vi "LEP_RV_BuildSpec_CommOptionsDlg.vi"(8 "error in (no error)":errorcluster, 10 "page sync rendezvous":T3, 11 "Close Event":refnum<user-event>) -> ()   [LabVIEW 2011]
doc: "Specifies TCP/IP options."
uses:
  resource/dialog/PreferencesDialog/optionsFrame_EventData1.ctl
  resource/dialog/PreferencesDialog/optionsFrame_PageInitData.ctl
  <vilib>/Platform/EmbProject/Plugins/utilities/LEP_Utilities_GetSetProjectData_Variant.vi
  <vilib>/Platform/EmbProject/Plugins/utilities/LEP_Utilities_GetSetProjectData_U32.vi
panel:
  out "Build settings conflicts":i32(listbox)=1
  in  "Target serial port":u16(ring) items=["0", "1", "2", "3"]
  in  "Console output":T1(radio)
  in  "MAC in target memory":bool
  in  "Secondary DNS":string
  in  "Primary DNS":string
  in  "MAC address":string
  in  "Target name":string
  in  "Gateway":string
  in  "Subnet mask":string
  in  "IP address":string
  in  "Use DHCP":bool
  in  "Page VI Init Data":T2
  in  "error msg format string":string="There was a problem applying the options from the %s category. The error message is \"%s.\""
  # "Console Output"
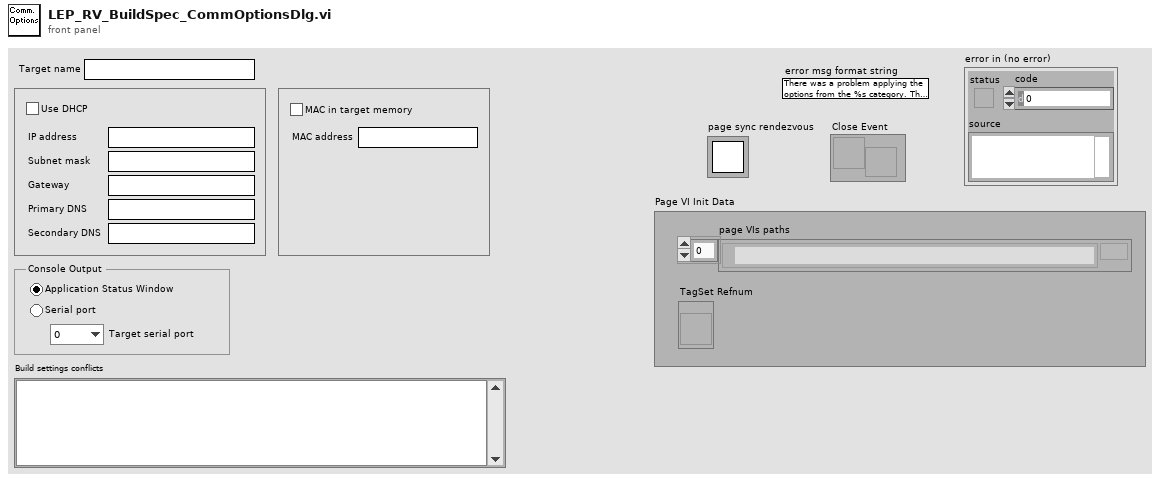
[diagram p1: front panel]
types:
  T1 = enum32{"Application Status Window", "Serial port"}
  T2 = typedef "optionsFrame_PageInitData.ctl" = cluster{"page VIs paths":path[], "TagSet Refnum":refnum<vi>}
  T3 = typedef "Rendezvous RefNum" = refnum<k1>
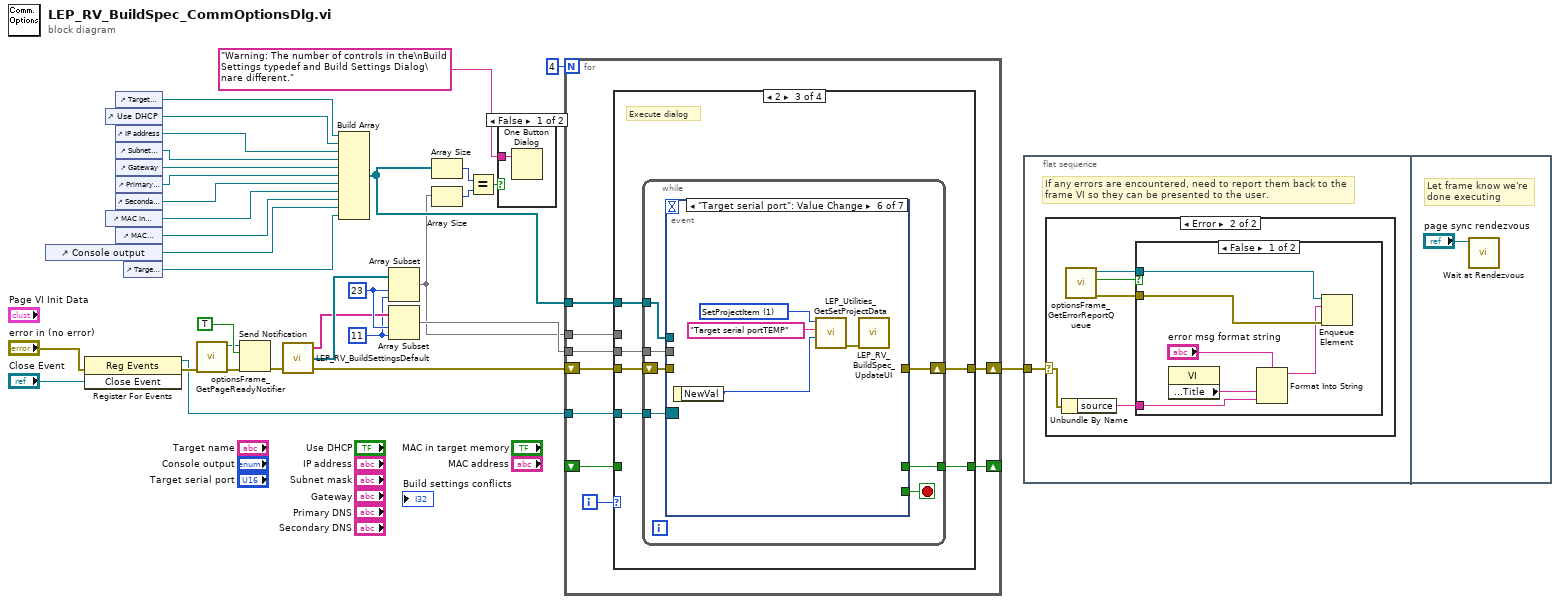
[diagram p0: block diagram]
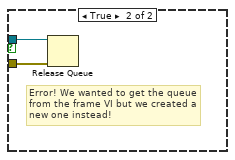
[diagram p3: hidden frame]
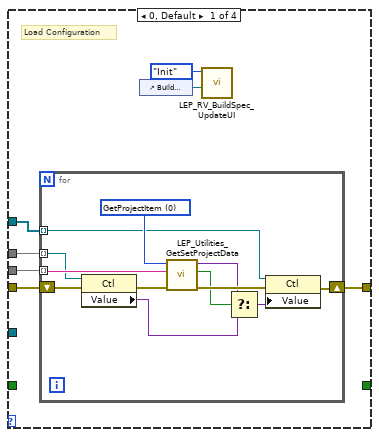
[diagram p5: hidden frame]
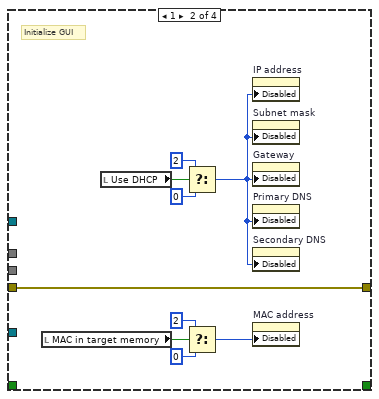
[diagram p6: hidden frame]
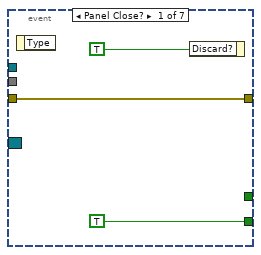
[diagram p7: hidden frame]
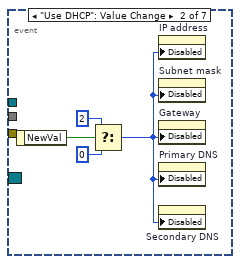
[diagram p8: hidden frame]
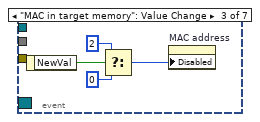
[diagram p9: hidden frame]
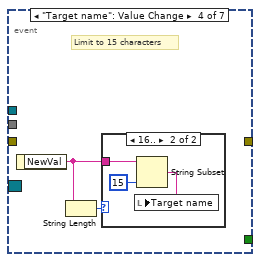
[diagram p10: hidden frame]
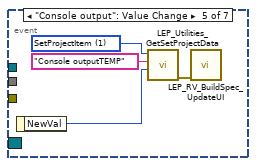
[diagram p12: hidden frame]
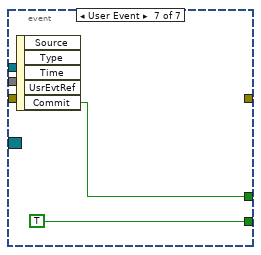
[diagram p13: hidden frame]
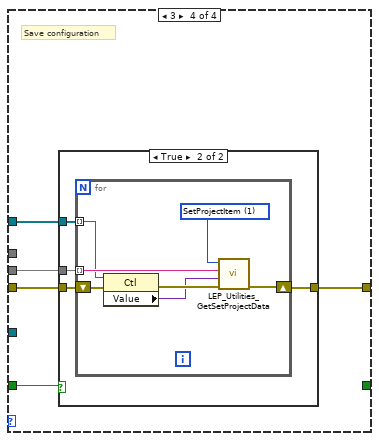
[diagram p14: hidden frame]
diagram:
  w1 = 11 ("length")
  w16 = 23 ("index")
  n1 = control-ref of="Console output"() -> (w2:refnum<vi>)
  n2 = register-events(error in="error in (no error)", "Close Event") -> (reference out=w19:refnum<event-registration>, error out=w22:errorcluster)  [unwired: 1 in]
  n3 = control-ref of="Use DHCP"() -> (w5:refnum<vi>)
  n4 = control-ref of="MAC in target memory"() -> (w9:refnum<vi>)
  n5 = control-ref of="Target name"() -> (w13:refnum<vi>)
  n6 = control-ref of="IP address"() -> (w6:refnum<vi>)
  n7 = control-ref of="Subnet mask"() -> (w7:refnum<vi>)
  n8 = control-ref of="Gateway"() -> (w8:refnum<vi>)
  n9 = control-ref of="Primary DNS"() -> (w12:refnum<vi>)
  n10 = control-ref of="Secondary DNS"() -> (w11:refnum<vi>)
  n11 = control-ref of="MAC address"() -> (w10:refnum<vi>)
  n12 = control-ref of="Target serial port"() -> (w3:refnum<vi>)
  n13 = call "optionsFrame_GetPageReadyNotifier.vi"("error in (no error)"=w22) -> ("error out"=w21:errorcluster, "notifier out"=w23:refnum<notifier>)  [unwired: 9 out]
  n14 = Send Notification(notification=TRUE, notifier=w23, error in (no error)=w21) -> (error out=w20:errorcluster)  [unwired: 1 out]
  n15 = call "LEP_RV_BuildSettingsDefault.vi"("error in (no error)"=w20) -> ("error out"=w32:errorcluster, "Default Values"=w17:refnum<vi>[], "Attribute Name"=w15:string[])  [unwired: 2 out]
  n16 = Build Array(w13, w5, w6, w7, w8, w12, w11, w9, w10, w2, w3) -> (w28:refnum<vi>[])
  n17 = Array Subset(array=w17, index=w16, length=w1) -> (w4:refnum<vi>[])
  n18 = Array Subset(array=w15, index=w16, length=w1) -> (w14:string[])
  n19 = Array Size(array=w28) -> (size(s)=w30:i32)
  n20 = Array Size(array=w4) -> (size(s)=w31:i32)
  n21 = Equal?(x=w30, y=w31) -> (x = y?=w29:bool)
  n22 = case shown="False" w29 {
    tunnel: "Warning: The number of controls in the\nBuild Settings typedef and Build Settings Dialog\nare different." -> [w34 _]
    frame False {
      n23 = One Button Dialog(message=w34) -> ()  [unwired: 2 out]
    }
    frame True {
    }
  }
  n24 = for {
    N: 4 -> [_]
    shift-right: [w41] -> w18
    shift-left: w32 -> [w42]
    shift-right: [w40] -> _
    shift-left: _ -> [w39]
    tunnel: w28 -> [w38]
    tunnel: w14 -> [w37]
    tunnel: w4 -> [w36]
    tunnel: w19 -> [w35]
    i -> [w43]
    n25 = case shown="2" w43 {
      tunnel: w42 -> [w49 w63 w77 w114]
      tunnel: [w48 w63 w76 w113] -> w41
      tunnel: [_ _ w75 _] -> w40
      tunnel: w39 -> [_ _ _ w115]
      tunnel: w38 -> [w50 _ w73 w111]
      tunnel: w37 -> [w47 _ w74 w112]
      tunnel: w36 -> [w46 _ _ _]
      tunnel: w35 -> [_ _ w72 _]
      frame 0, Default {
        # "Load Configuration"
        n26 = for {
          tunnel: w50 -> [w51] mode=indexing
          shift-right: [w60] -> w48
          shift-left: w49 -> [w58]
          tunnel: w47 -> [w59] mode=indexing
          tunnel: w46 -> [w56] mode=indexing
          w62 = u16 0 items=["GetProjectItem", "SetProjectItem"] ("Command")
          n27 = property class="Ctl"(reference=w56, error in=w58) -> (error out=w57:errorcluster, "Value"=w52:variant)  [unwired: 1 out]
          n28 = call-poly <vilib>:"LEP_Utilities_GetSetProjectData.vi"("error in"=w57, "ItemName"=w59, "Command"=w62) -> ("error out"=w61:errorcluster, "Found/Replaced?"=w53:bool, "Variant Out"=w54:variant)  [unwired: 2 in, 4 out]
          n29 = Select(t=w54, s=w53, f=w52) -> (s? t:f=w55:variant)
          n30 = property class="Ctl"(reference=w51, error in=w61, "Value"=w55) -> (error out=w60:errorcluster)  [unwired: 1 out]
        }
        n31 = control-ref of="Build settings conflicts"() -> (w44:refnum<vi>)
        n32 = call "LEP_RV_BuildSpec_UpdateUI.vi"("Build conflicts ref"=w44, "Action"=enum16{"Init", "UpdateUI"}."Init") -> ()  [unwired: 2 in, 8 out]
      }
      frame 1 {
        # "Initialize GUI"
        n33 = local read "MAC in target memory"() -> (w71:bool)
        n34 = local read "Use DHCP"() -> (w66:bool)
        n35 = Select(t=u8 2 ("Disabled"), s=w66, f=u8 0 ("Disabled")) -> (s? t:f=w64:u8)
        n36 = Select(t=u8 2 ("Disabled"), s=w71, f=u8 0 ("Disabled")) -> (s? t:f=w65:u8)
        n37 = property on="IP address" class="Str"("Disabled"=w64) -> ()  [unwired: 2 in, 2 out]
        n38 = property on="Subnet mask" class="Str"("Disabled"=w64) -> ()  [unwired: 2 in, 2 out]
        n39 = property on="Gateway" class="Str"("Disabled"=w64) -> ()  [unwired: 2 in, 2 out]
        n40 = property on="Primary DNS" class="Str"("Disabled"=w64) -> ()  [unwired: 2 in, 2 out]
        n41 = property on="Secondary DNS" class="Str"("Disabled"=w64) -> ()  [unwired: 2 in, 2 out]
        n42 = property on="MAC address" class="Str"("Disabled"=w65) -> ()  [unwired: 2 in, 2 out]
      }
      frame 2 {
        # "Execute dialog"
        n43 = while {
          shift-right: [w83] -> w76
          shift-left: w77 -> [w84]
          tunnel: [w82] -> w75
          tunnel: w74 -> [w80]
          tunnel: w73 -> [w79]
          tunnel: w72 -> [w78]
          stop <- w81 stop-if-true
          n44 = event shown="[5] \"Target serial port\": Value Change" {
            selector: w78 -> [_ _ _ _ _ _ _]
            dyn-events: _ -> [_ _ _ _ _ _ _]
            timeout: _ -> [_ _ _ _ _ _ _]
            tunnel: w84 -> [w86 _ _ _ _ _ _]
            tunnel: [w86 _ _ _ _ _ _] -> w83
            tunnel: [_ _ _ _ _ _ w109] -> w82
            tunnel: [TRUE _ _ _ _ _ TRUE ("Cancel")] -> w81
            tunnel: w80 -> [_ _ _ _ _ _ _]
            tunnel: w79 -> [_ _ _ _ _ _ _]
            event Panel Close? {
              n45 = event-data() -> ()  [unwired: 2 out]
              n46 = event-data("Discard?"=TRUE) -> ()  [unwired: 1 in, 1 out]
            }
            event "Use DHCP": Value Change {
              n47 = event-data() -> ("NewVal"=w88:bool)  [unwired: 1 out]
              n48 = Select(t=u8 2 ("Disabled"), s=w88, f=u8 0 ("Disabled")) -> (s? t:f=w89:u8)
              n49 = property on="IP address" class="Str"("Disabled"=w89) -> ()  [unwired: 2 in, 2 out]
              n50 = property on="Subnet mask" class="Str"("Disabled"=w89) -> ()  [unwired: 2 in, 2 out]
              n51 = property on="Gateway" class="Str"("Disabled"=w89) -> ()  [unwired: 2 in, 2 out]
              n52 = property on="Primary DNS" class="Str"("Disabled"=w89) -> ()  [unwired: 2 in, 2 out]
              n53 = property on="Secondary DNS" class="Str"("Disabled"=w89) -> ()  [unwired: 2 in, 2 out]
            }
            event "MAC in target memory": Value Change {
              n54 = event-data() -> ("NewVal"=w92:bool)  [unwired: 1 out]
              n55 = Select(t=u8 2 ("Disabled"), s=w92, f=u8 0 ("Disabled")) -> (s? t:f=w93:u8)
              n56 = property on="MAC address" class="Str"("Disabled"=w93) -> ()  [unwired: 2 in, 2 out]
            }
            event "Target name": Value Change {
              # "Limit to 15 characters"
              n57 = event-data() -> ("NewVal"=w96:string)  [unwired: 1 out]
              n58 = String Length(string=w96) -> (length=w97:i32)
              n59 = case shown="16.." w97 {
                tunnel: w96 -> [_ w100]
                frame Default {
                }
                frame 16.. {
                  n60 = String Subset(string=w100, length (rest)=15 ("length (rest)")) -> (substring=w98:string)  [unwired: 1 out]
                  n61 = local write "Target name"(w98) -> ()
                }
              }
            }
            event "Console output": Value Change {
              w101 = u16 1 items=["GetProjectItem", "SetProjectItem"] ("Command")
              n62 = event-data() -> ("NewVal"=w102:T1)  [unwired: 1 out]
              n63 = call-poly <vilib>:"LEP_Utilities_GetSetProjectData.vi"("data in"=w102, "ItemName"="Console outputTEMP", "Command"=w101) -> ("error out"=w104:errorcluster)  [unwired: 2 in, 6 out]
              n64 = call "LEP_RV_BuildSpec_UpdateUI.vi"("error in (no error)"=w104) -> ()  [unwired: 3 in, 8 out]
            }
            event "Target serial port": Value Change {
              w107 = u16 1 items=["GetProjectItem", "SetProjectItem"] ("Command")
              n65 = event-data() -> ("NewVal"=w106:u16)  [unwired: 1 out]
              n66 = call-poly <vilib>:"LEP_Utilities_GetSetProjectData.vi"("data in"=w106, "ItemName"="Target serial portTEMP", "Command"=w107) -> ("error out"=w108:errorcluster)  [unwired: 2 in, 6 out]
              n67 = call "LEP_RV_BuildSpec_UpdateUI.vi"("error in (no error)"=w108) -> ()  [unwired: 3 in, 8 out]
            }
            event User Event {
              n68 = event-data() -> ("Commit"=w109:bool)  [unwired: 5 out]
            }
          }
        }
      }
      frame 3 {
        # "Save configuration"
        n69 = case shown="True" w115 {
          tunnel: w114 -> [w116 w120]
          tunnel: [w116 w117] -> w113
          tunnel: w112 -> [_ w119]
          tunnel: w111 -> [_ w118]
          frame False {
          }
          frame True {
            n70 = for {
              shift-right: [w122] -> w117
              shift-left: w120 -> [w126]
              tunnel: w119 -> [w124] mode=indexing
              tunnel: w118 -> [w121] mode=indexing
              w127 = u16 1 items=["GetProjectItem", "SetProjectItem"] ("Command")
              n71 = property class="Ctl"(reference=w121, error in=w126) -> (error out=w125:errorcluster, "Value"=w123:variant)  [unwired: 1 out]
              n72 = call-poly <vilib>:"LEP_Utilities_GetSetProjectData.vi"("error in"=w125, "Variant In"=w123, "ItemName"=w124, "Command"=w127) -> ("error out"=w122:errorcluster)  [unwired: 1 in, 6 out]
            }
          }
        }
      }
    }
  }
  n73 = flat-sequence {
    tunnel: w18 -> [w128]
    frame #0 {
      # "If any errors are encountered, need to report them back to the \nframe VI so they can be presented to the user."
      n74 = case shown="Error" w128 {
        selector: w128 -> [_ w130]
        frame No Error {
        }
        frame Error {
          n75 = Unbundle By Name(w130) -> ("source"=w129:string)
          n76 = call "optionsFrame_GetErrorReportQueue.vi"() -> ("error out"=w131:errorcluster, "created new?"=w133:bool, "queue out"=w132:refnum<queue>)  [unwired: 9 out]
          n77 = case shown="False" w133 {
            tunnel: w132 -> [w139 w141]
            tunnel: w131 -> [w138 w140]
            tunnel: w129 -> [w135 _]
            frame False {
              n78 = property class="VI"() -> ("Front Panel.Title"=w136:string)  [unwired: 2 in, 2 out]
              n79 = Format Into String(format string="error msg format string", w136, w135) -> (resulting string=w134:string)  [unwired: 2 in, 1 out]
              n80 = Enqueue Element(queue=w139, element=w134, error in (no error)=w138) -> ()  [unwired: 4 out]
            }
            frame True {
              # "Error! We wanted to get the queue\nfrom the frame VI but we created a\nnew one instead!"
              n81 = Release Queue(queue=w141, error in (no error)=w140) -> ()  [unwired: 4 out]
            }
          }
        }
      }
    }
    frame #1 {
      # "Let frame know we're \ndone executing"
      n82 = call <vilib>:"Wait at Rendezvous.vi"("rendezvous"="page sync rendezvous") -> ()  [unwired: 2 in, 5 out]
    }
  }
